vi "Main.vi"(11 "Module Admin":refnum<class "Delacor_lib_QMH_Module Admin.lvclass">) -> ()   [LabVIEW 2024, in "PLC.lvlib"]
doc: "This template is based off of the Queued Message Handler design pattern and the Queued Message Handler project template that ships with LabVIEW.\n\nThe main difference is that the queue is private to this module and communication between modules is performed via Broadcast and Request events.\n\nRequest events are wrapped in public API methods and are handled in the Event Handling Loop (EHL) of this VI. Any module can register for Broadcast events sent by this module. The EHL generates messages based on user interface actions.\n\nThe Message Handling Loop (MHL) processes messages generated by the EHL, or by other messages. The messages are string values, so new messages can be added easily to the Message Cases case structure in the MHL. Each message cluster can also provide an optional value for Message Data, which is a variant that can be converted to whatever message-specific data is required.\n_____\nBased on DQMH Dev Tools: Project Template 7.1.0.1503."
uses:
  PLC.lvlib
  <vilib>/Delacor/Delacor QMH/Libraries/Module Admin_class/Delacor_lib_QMH_Module Admin.lvclass
  Module Data--cluster.ctl
  <vilib>/Delacor/Delacor QMH/Libraries/Message Queue_class/Delacor_lib_QMH_Message Queue.lvclass/Delacor_lib_QMH_Message Queue.ctl
  Stop Argument--cluster.ctl
  <vilib>/Delacor/Delacor QMH/Libraries/Module Admin_class/Delacor_lib_QMH_Module Admin.lvclass/Delacor_lib_QMH_Module Admin.ctl
  set coil value Argument--cluster.ctl
  set register value Argument--cluster.ctl
  read coils Argument--cluster.ctl
  connect Argument--cluster.ctl
  <vilib>/Utility/miscctls.llb/LVPointTypeDef.ctl
  GUI/Controls/HW Modules.ctl
  <vilib>/Delacor/Delacor QMH/Libraries/Message Queue_class/Delacor_lib_QMH_Enqueue Message (Single).vi
  <vilib>/Delacor/Delacor QMH/Libraries/Module Admin_class/Delacor_lib_QMH_Get External Launch.vi
  <vilib>/NI/Modbus Library/API/Wrapper/Create TCP Master.vi
  <vilib>/Delacor/Delacor QMH/Libraries/Message Queue_class/Delacor_lib_QMH_Message Queue.lvclass
  <vilib>/NI/Modbus Library/API/Master/Modbus Master.lvclass
  <vilib>/NI/Modbus Library/API/Wrapper/API Main.lvlib
  GUI/GUI.lvlib
  Controller/Controller.lvlib
panel:
  out "coils":bool[](array[boolean])
  out "error out":errorcluster
  out "Status":string
  in  "Simulate MHL Error":bool
  in  "Simulate EHL Error":bool
  # "Other processes communicate with this Module via its Public API (wrappers for its Request Events).\n\nThis Module communicates with other processes via its Broadcast Events.\nAny process that wants to receive these messages can register for this module's Broadcast events."
  # "This template is for the DQMH framework. See the block diagram for more information on how to use this template."
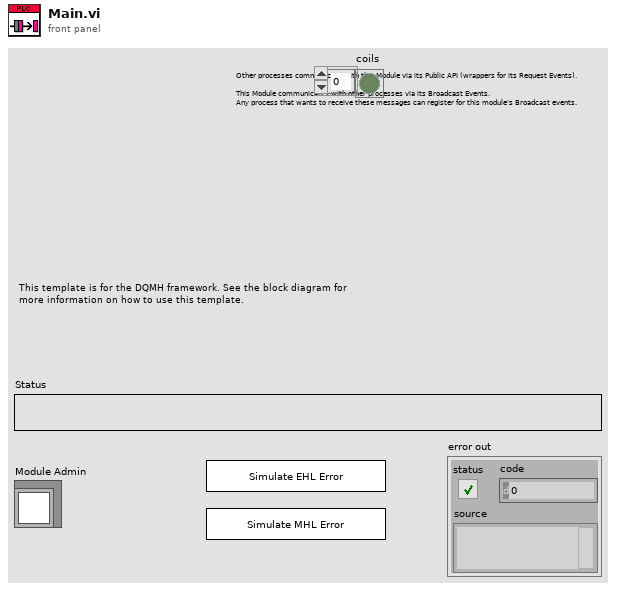
[diagram p1: front panel]
types:
  T1 = typedef "PLC.lvlib/Request Events--cluster.ctl" = cluster{"Stop Module":refnum<user-event>, "Show Panel":refnum<user-event>, "Hide Panel":refnum<user-event>, "Get Module Execution Status":refnum<user-event>, "Show Diagram":refnum<user-event>, "set coil value":refnum<user-event>, "set register value":refnum<user-event>, "Private.read coils":refnum<user-event>, "connect":refnum<user-event>}
  T2 = typedef "PLC.lvlib/Module Data--cluster.ctl" = cluster{"Status":string}
  T3 = enum32{"invalid lock state", "Not Locked", "Locked (No Password)", "Password-protected"}
  T4 = typedef "PLC.lvlib/Stop Argument--cluster.ctl" = cluster{"Origin":string, "Exit via Stop Module Req?":bool, "Wait for Module to stop?":bool}
  T5 = typedef "PLC.lvlib/set coil value Argument--cluster.ctl" = cluster{"ON/OFF":bool, "Ring":u16}
  T6 = typedef "PLC.lvlib/set register value Argument--cluster.ctl" = cluster{"Register number":u16, "value":dbl}
  T7 = typedef "PLC.lvlib/read coils Argument--cluster.ctl" = cluster{"number of coils to read":dbl}
  T8 = typedef "PLC.lvlib/connect Argument--cluster.ctl" = cluster{"IP address":string, "Port":dbl, "Flush events":bool}
  T9 = typedef "LVPointTypeDef.ctl" = cluster{"Horizontal":i16, "Vertical":i16}
  T10 = enum32{"Invalid", "Standard", "Closed", "Hidden", "Minimized", "Maximized"}
  T11 = typedef "HW Modules.ctl" = string
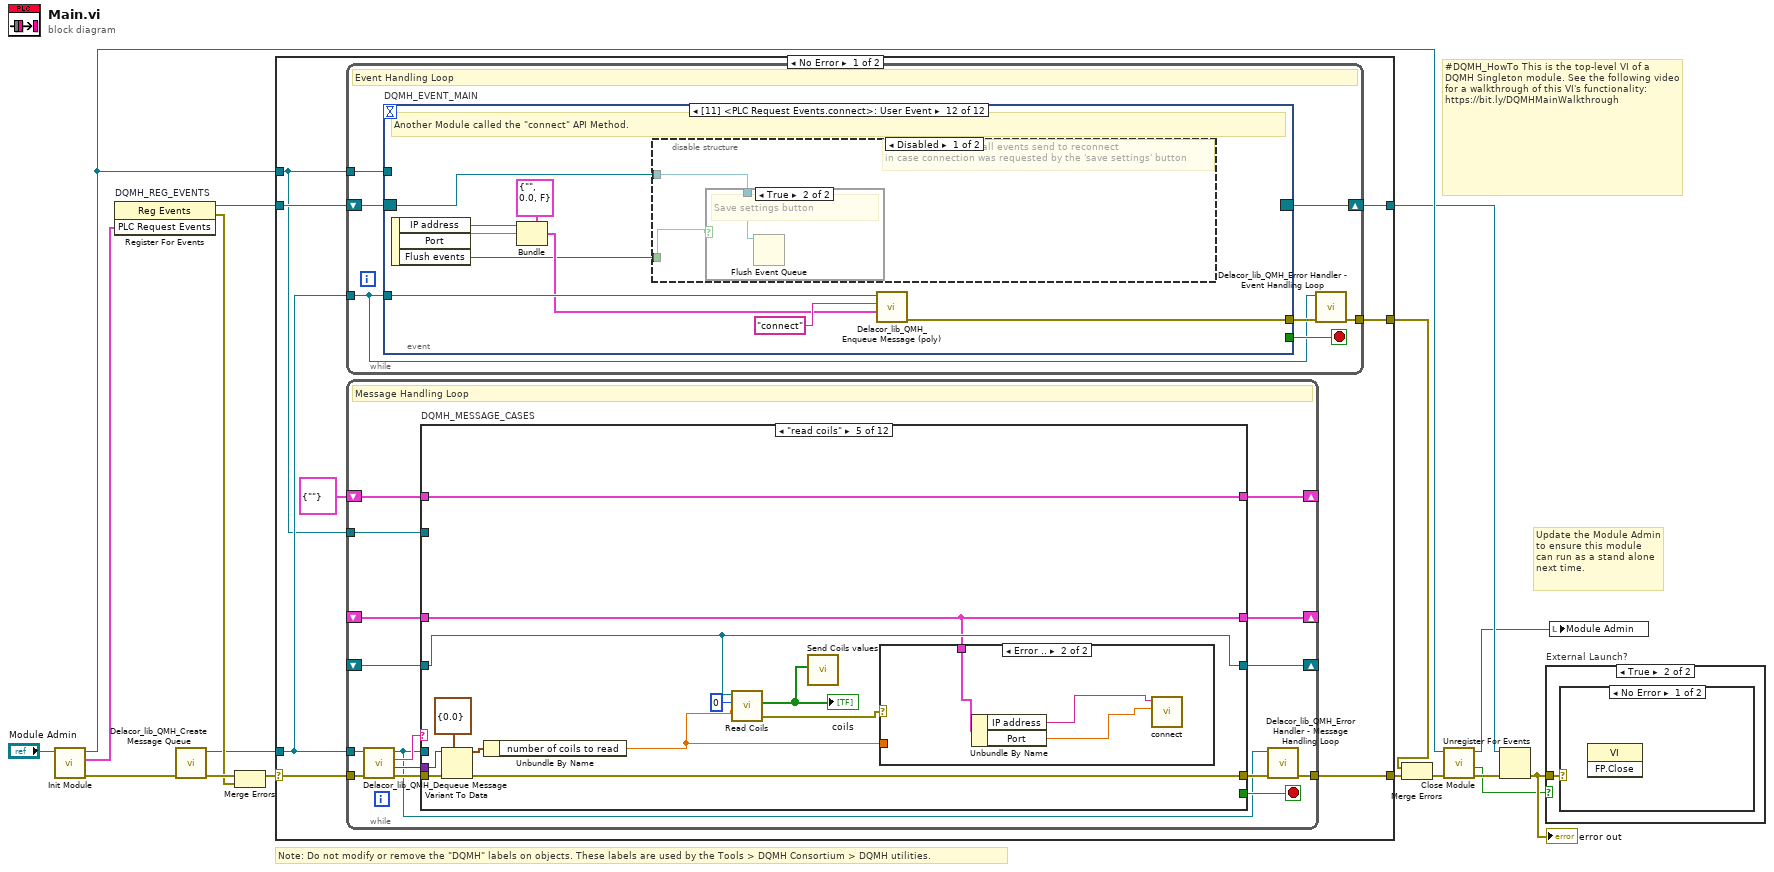
[diagram p0: block diagram]
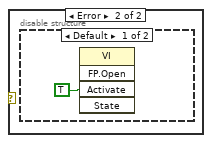
[diagram p3: hidden frame]
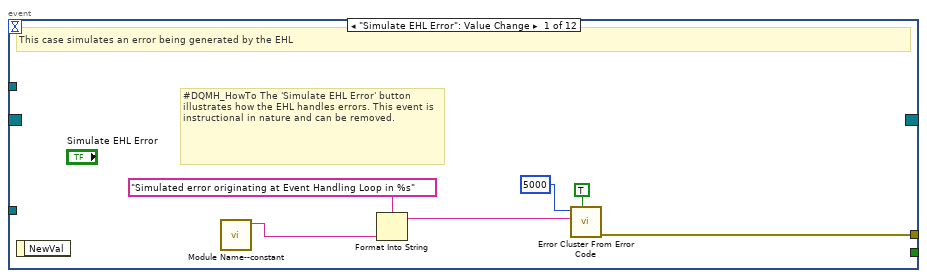
[diagram p5: hidden frame]
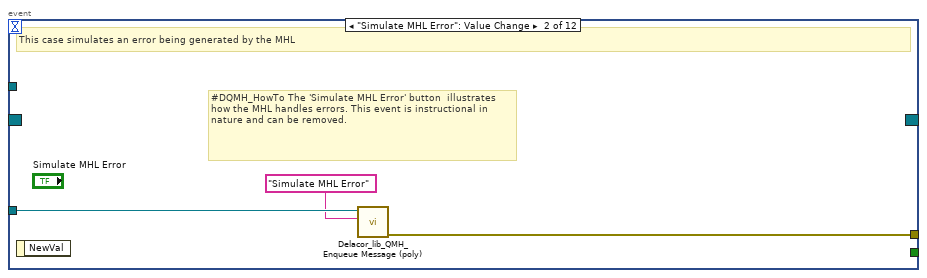
[diagram p6: hidden frame]
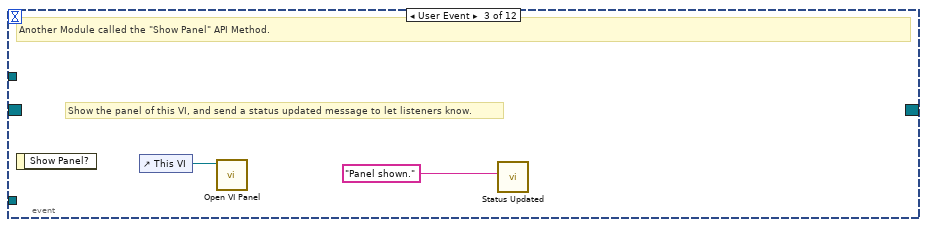
[diagram p7: hidden frame]
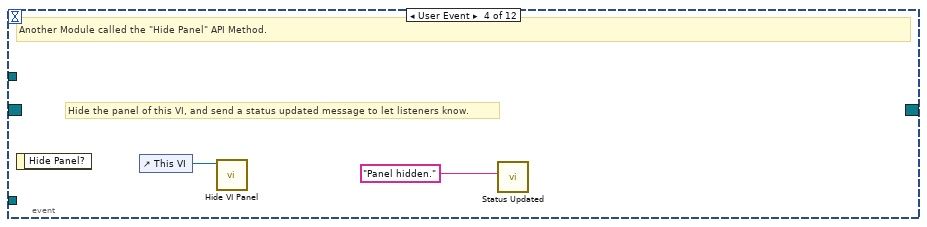
[diagram p8: hidden frame]
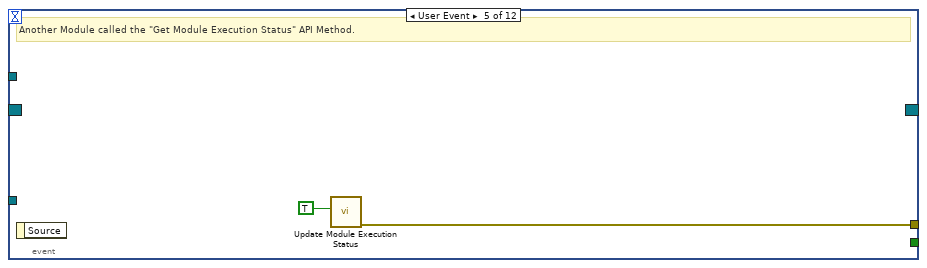
[diagram p9: hidden frame]
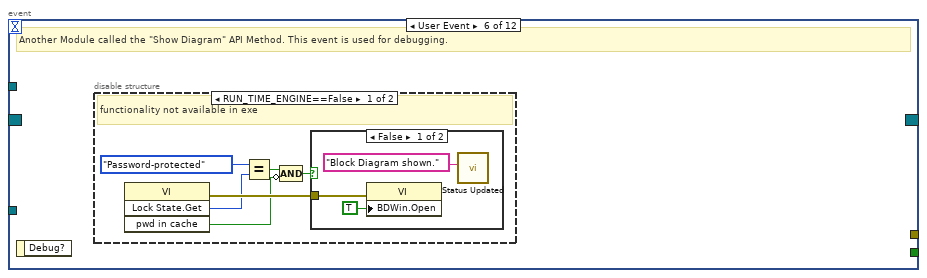
[diagram p10: hidden frame]
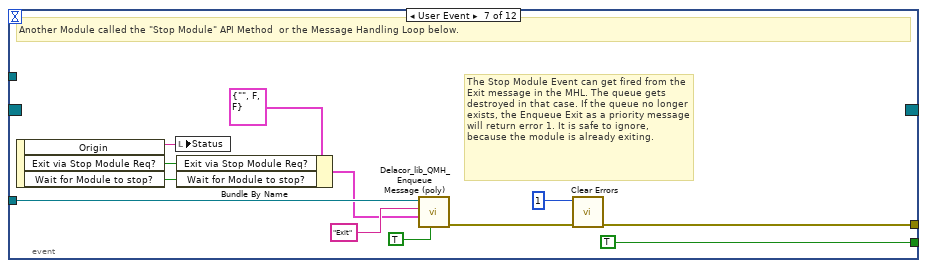
[diagram p13: hidden frame]
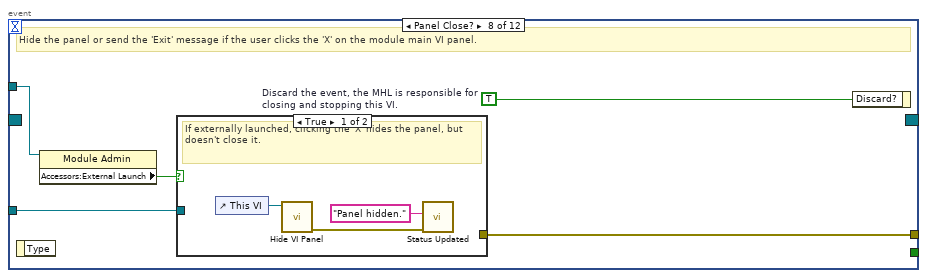
[diagram p14: hidden frame]
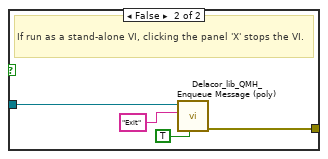
[diagram p15: hidden frame]
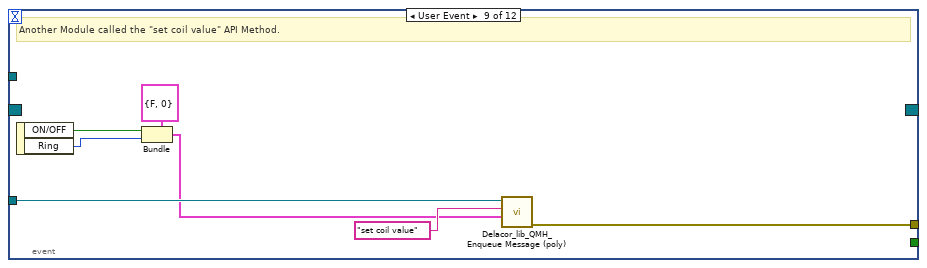
[diagram p16: hidden frame]
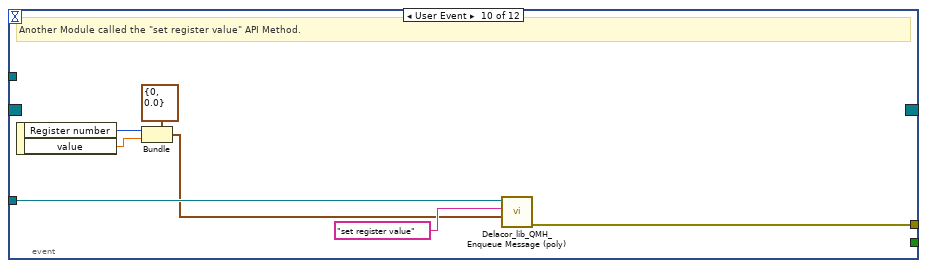
[diagram p17: hidden frame]
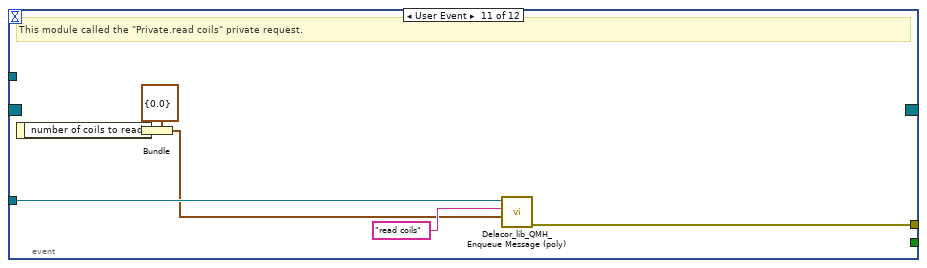
[diagram p18: hidden frame]
diagram:
  # "#DQMH_HowTo This is the top-level VI of a DQMH Singleton module. See the following video for a walkthrough of this VI's functionality: https://bit.ly/DQMHMainWalkthrough"
  # "Note: Do not modify or remove the \"DQMH\" labels on objects. These labels are used by the Tools > DQMH Consortium > DQMH utilities."
  # "Update the Module Admin to ensure this module can run as a stand alone next time."
  n1 = call "Init Module.vi"("Singleton Module Admin in"="Module Admin") -> ("error out"=w16:errorcluster, "PLC Request Events"=w5:T1, "Singleton Module Admin out"=w8:refnum<class "Delacor_lib_QMH_Module Admin.lvclass">)  [unwired: 8 in]
  n2 = register-events "DQMH_REG_EVENTS"(w5) -> (reference out=w6:refnum<event-registration>, error out=w9:errorcluster)  [unwired: 2 in]
  n3 = call <vilib>:"Delacor_lib_QMH_Create Message Queue.vi"("error in"=w16) -> ("error out"=w11:errorcluster, "Message Queue"=w4:refnum<class "Delacor_lib_QMH_Message Queue.lvclass">)  [unwired: 9 in]
  n4 = Merge Errors(w11, w9) -> (w10:errorcluster)
  n5 = case shown="No Error" w10 {
    selector: w10 -> [w23 w292]
    tunnel: [w25 w291] -> w17
    tunnel: [w22 w290] -> w7
    tunnel: w6 -> [w20 w290]
    tunnel: w4 -> [w19 w285]
    tunnel: [w24 _] -> w14
    tunnel: w8 -> [w18 w286]
    frame No Error {
      n6 = while {
        tunnel: w19 -> [w26]
        shift-right: [w29] -> w22
        shift-left: w20 -> [w30]
        tunnel: [w31] -> w24
        tunnel: w18 -> [w27]
        stop <- w28 stop-if-true
        # "Event Handling Loop"
        n7 = event "DQMH_EVENT_MAIN" shown="[11] <PLC Request Events.connect>: User Event" {
          selector: w30 -> [_ _ _ _ _ _ _ _ _ _ _ w102]
          dyn-events: [_ _ _ _ _ _ _ _ _ _ _ _] -> w29
          timeout: _ -> [_ _ _ _ _ _ _ _ _ _ _ _]
          tunnel: [_ _ _ _ _ _ TRUE ("Discard?") _ _ _ _ _] -> w28
          tunnel: w26 -> [_ w40 _ _ _ _ w64 w71 w87 w94 w100 w109]
          tunnel: [w38 w41 _ _ w47 _ w67 w73 w81 w88 w95 w103] -> w32
          tunnel: w27 -> [_ _ _ _ _ _ _ w70 _ _ _ _]
          event "Simulate EHL Error": Value Change {
            # "#DQMH_HowTo The 'Simulate EHL Error' button  illustrates how the EHL handles errors. This event is instructional in nature and can be removed."
            # "This case simulates an error being generated by the EHL"
            n8 = event-data() -> ()  [unwired: 1 in, 1 out]
            n9 = call "Module Name--constant.vi"() -> ("Module Name"=w35:string)  [unwired: 11 in]
            n10 = Format Into String(format string="Simulated error originating at Event Handling Loop in %s", w35) -> (resulting string=w36:string)  [unwired: 2 in, 1 out]
            n11 = call <vilib>:"Error Cluster From Error Code.vi"("show call chain? (False)"=TRUE, "error message (\"\")"=w36, "error code (0)"=5000) -> ("error out"=w38:errorcluster)  [unwired: 6 in]
          }
          event "Simulate MHL Error": Value Change {
            # "#DQMH_HowTo The 'Simulate MHL Error' button  illustrates how the MHL handles errors. This event is instructional in nature and can be removed."
            # "This case simulates an error being generated by the MHL"
            n12 = event-data() -> ()  [unwired: 1 in, 1 out]
            n13 = call-poly <vilib>:"Delacor_lib_QMH_Enqueue Message (poly).vi"("Message"="Simulate MHL Error", "Message Queue in"=w40) -> ("error out"=w41:errorcluster)  [unwired: 8 in, 1 out]
          }
          event User Event {
            # "Show the panel of this VI, and send a status updated message to let listeners know."
            # "Another Module called the \"Show Panel\" API Method."
            n14 = event-data() -> ()  [unwired: 1 in, 1 out]
            n15 = control-ref of="This VI"() -> (w43:refnum<vi>)
            n16 = call "Open VI Panel.vi"("VI"=w43) -> ()  [unwired: 10 in, 1 out]
            n17 = call "Status Updated.vi"("Status"="Panel shown." ("format string")) -> ()  [unwired: 10 in, 1 out]
          }
          event User Event {
            # "Hide the panel of this VI, and send a status updated message to let listeners know."
            # "Another Module called the \"Hide Panel\" API Method."
            n18 = event-data() -> ()  [unwired: 1 in, 1 out]
            n19 = control-ref of="This VI"() -> (w45:refnum<vi>)
            n20 = call "Hide VI Panel.vi"("VI"=w45) -> ()  [unwired: 10 in, 1 out]
            n21 = call "Status Updated.vi"("Status"="Panel hidden." ("format string")) -> ()  [unwired: 10 in, 1 out]
          }
          event User Event {
            # "Another Module called the \"Get Module Execution Status\" API Method."
            n22 = event-data() -> ()  [unwired: 1 in, 1 out]
            n23 = call "Update Module Execution Status.vi"("Running?"=TRUE) -> ("error out"=w47:errorcluster)  [unwired: 10 in]
          }
          event User Event {
            # "Another Module called the \"Show Diagram\" API Method. This event is used for debugging."
            n24 = event-data() -> ()  [unwired: 1 in, 1 out]
            n25 = disable-structure shown="RUN_TIME_ENGINE==False" {
              frame condition #0 (active) {
                # "functionality not available in exe"
                n26 = invoke on="Invoke Node" class="VI" method="Lock State.Get"() -> (error out=w53:errorcluster, "Get Lock State"=w52:T3, "pwd in cache"=w49:bool)  [unwired: 4 in, 1 out]
                n27 = Equal?(x=T3."Password-protected", y=w52) -> (x = y?=w50:bool)
                n28 = Compound Arithmetic op=AND(w50, invert w49) -> (w48:bool)
                n29 = case shown="False" w48 {
                  tunnel: w53 -> [w56 _]
                  frame False {
                    n30 = property on="Property Node" class="VI"(error in=w56, "BDWin.Open"=TRUE ("Block Diagram Window:Open")) -> ()  [unwired: 1 in, 2 out]
                    n31 = call "Status Updated.vi"("Status"="Block Diagram shown." ("format string")) -> ()  [unwired: 10 in, 1 out]
                  }
                  frame True {
                    # "Password-protected VI, and the password is not in the cache. Do not show the diagram."
                  }
                }
              }
              frame condition #1 {
              }
            }
          }
          event User Event {
            # "The Stop Module Event can get fired from the Exit message in the MHL. The queue gets destroyed in that case. If the queue no longer exists, the Enqueue Exit as a priority message will return error 1. It is safe to ignore, because the module is already exiting."
            # "Another Module called the \"Stop Module\" API Method  or the Message Handling Loop below."
            n32 = event-data() -> ("Origin"=w63:string, "Exit via Stop Module Req?"=w59:bool, "Wait for Module to stop?"=w58:bool)  [unwired: 1 in]
            n33 = local write "Status"(w63) -> ()
            n34 = Bundle By Name(cluster=T4 {"Origin"="", "Exit via Stop Module Req?"=FALSE, "Wait for Module to stop?"=FALSE} ("Stop Argument"), "Exit via Stop Module Req?"=w59, "Wait for Module to stop?"=w58) -> (w57:T4)
            n35 = call-poly <vilib>:"Delacor_lib_QMH_Enqueue Message (poly).vi"("Priority Message? (F)"=TRUE, "Message Data"=w57, "Message"="Exit", "Message Queue in"=w64) -> ("error out"=w68:errorcluster)  [unwired: 6 in, 1 out]
            n36 = call <vilib>:"Clear Errors.vi"("error in (no error)"=w68, "specific error code to clear (0: all)"=1) -> ("error out"=w67:errorcluster)  [unwired: 4 in, 1 out]
          }
          event Panel Close? {
            w72 = TRUE  # Discard the event, the MHL is responsible for closing and stopping this VI.
            # "Hide the panel or send the 'Exit' message if the user clicks the 'X' on the module main VI panel."
            n37 = event-data() -> ()  [unwired: 1 in, 1 out]
            n38 = property on="Property Node" class="Module Admin"(reference=w70) -> ("Accessors:External Launch"=w69:bool)  [unwired: 1 in, 2 out]
            n39 = case shown="True" w69 {
              tunnel: w71 -> [_ w79]
              tunnel: [_ w80] -> w73
              frame True {
                # "If externally launched, clicking the 'X' hides the panel, but doesn't close it."
                n40 = control-ref of="This VI"() -> (w76:refnum<vi>)
                n41 = call "Hide VI Panel.vi"("VI"=w76) -> ("error out"=w74:errorcluster)  [unwired: 10 in]
                n42 = call "Status Updated.vi"("error in"=w74, "Status"="Panel hidden." ("format string")) -> ()  [unwired: 9 in, 1 out]
              }
              frame False {
                # "If run as a stand-alone VI, clicking the panel 'X' stops the VI."
                n43 = call-poly <vilib>:"Delacor_lib_QMH_Enqueue Message (poly).vi"("Priority Message? (F)"=TRUE, "Message"="Exit", "Message Queue in"=w79) -> ("error out"=w80:errorcluster)  [unwired: 7 in, 1 out]
              }
            }
            n44 = event-data ("Event Filter Node")("Discard?"=w72) -> ()  [unwired: 1 in, 1 out]
          }
          event User Event {
            # "Another Module called the \"set coil value\" API Method."
            n45 = event-data() -> ("ON/OFF"=w83:bool, "Ring"=w82:u16)  [unwired: 1 in]
            n46 = Bundle(cluster=T5 {"ON/OFF"=FALSE, "Ring"=0} ("set coil value Argument"), "ON/OFF"=w83, "Ring"=w82) -> (w84:T5)
            n47 = call-poly <vilib>:"Delacor_lib_QMH_Enqueue Message (poly).vi"("Message Data"=w84, "Message"="set coil value", "Message Queue in"=w87) -> ("error out"=w81:errorcluster)  [unwired: 7 in, 1 out]
          }
          event User Event {
            # "Another Module called the \"set register value\" API Method."
            n48 = event-data() -> ("Register number"=w90:u16, "value"=w89:dbl)  [unwired: 1 in]
            n49 = Bundle(cluster=T6 {"Register number"=0, "value"=0.0} ("set register value Argument"), "Register number"=w90, "value"=w89) -> (w91:T6)
            n50 = call-poly <vilib>:"Delacor_lib_QMH_Enqueue Message (poly).vi"("Message Data"=w91, "Message"="set register value", "Message Queue in"=w94) -> ("error out"=w88:errorcluster)  [unwired: 7 in, 1 out]
          }
          event User Event {
            # "This module called the \"Private.read coils\" private request."
            n51 = event-data() -> ("number of coils to read"=w96:dbl)  [unwired: 1 in]
            n52 = Bundle(cluster=T7 {"number of coils to read"=0.0} ("read coils Argument"), "number of coils to read"=w96) -> (w97:T7)
            n53 = call-poly <vilib>:"Delacor_lib_QMH_Enqueue Message (poly).vi"("Message Data"=w97, "Message"="read coils", "Message Queue in"=w100) -> ("error out"=w95:errorcluster)  [unwired: 7 in, 1 out]
          }
          event User Event {
            # "Another Module called the \"connect\" API Method."
            n54 = event-data() -> ("IP address"=w105:string, "Port"=w104:dbl, "Flush events"=w101:bool)  [unwired: 1 in]
            n55 = Bundle(cluster=T8 {"IP address"="", "Port"=0.0, "Flush events"=FALSE} ("connect Argument"), "IP address"=w105, "Port"=w104) -> (w106:T8)  [unwired: 1 in]
            n56 = disable-structure shown="Disabled" {
              disable-tunnel: w102 -> [w111 _]
              disable-tunnel: w101 -> [w110 _]
              frame Disabled {
                # "this is used to flush all events send to reconnect\nin case connection was requested by the 'save settings' button"
                n57 = case shown="True" w110 {
                  tunnel: w111 -> [_ w112]
                  frame False {
                    # "reconnect by the same module"
                  }
                  frame True {
                    # "Save settings button"
                    n58 = Flush Event Queue(0:w112) -> ()  [unwired: 5 in, 3 out]
                  }
                }
              }
              frame Enabled {
              }
            }
            n59 = call-poly <vilib>:"Delacor_lib_QMH_Enqueue Message (poly).vi"("Message Data"=w106, "Message"="connect", "Message Queue in"=w109) -> ("error out"=w103:errorcluster)  [unwired: 7 in, 1 out]
          }
        }
        n60 = call-dynamic "Delacor_lib_QMH_Error Handler - Event Handling Loop.vi"("error in"=w32, "Message Queue in"=w26) -> ("dup error in"=w31:errorcluster)  [unwired: 8 in, 1 out]
      }
      n61 = while {
        tunnel: w19 -> [w117]
        shift-right: [w125] -> _
        shift-left: T2 {"Status"=""} ("Data Cluster") -> [w126]
        tunnel: w23 -> [w128]
        tunnel: [w120] -> w25
        tunnel: w18 -> [w121]
        shift-right: [w116] -> _
        shift-left: _ -> [w115]
        shift-right: [w114] -> _
        shift-left: _ -> [w113]
        stop <- w124 stop-if-true
        # "Message Handling Loop"
        n62 = call-dynamic "Delacor_lib_QMH_Dequeue Message.vi"("error in"=w128, "Message Queue in"=w117) -> ("error out"=w127:errorcluster, "Message Data"=w122:variant, "Message"=w123:string, "Message Queue out"=w118:refnum<class "Delacor_lib_QMH_Message Queue.lvclass">)  [unwired: 6 in]
        n63 = case "DQMH_MESSAGE_CASES" shown="\"read coils\"" w123 {
          selector: w123 -> [_ _ _ _ _ _ _ _ _ _ _ w280]
          tunnel: w118 -> [_ _ _ _ _ w189 _ _ _ w242 w266 _]
          tunnel: w127 -> [w148 w154 w162 w170 w182 w205 w221 w225 w236 w249 w272 w283]
          tunnel: [w146 w154 w160 w168 w180 w203 w220 w225 w235 w245 w267 w284] -> w119
          tunnel: w126 -> [w137 w153 w161 w169 w181 w204 w219 w224 w233 w244 w265 w281]
          tunnel: [w136 w153 w161 w169 w181 w204 w219 w224 w233 w244 w265 w281] -> w125
          tunnel: [_ _ _ _ _ _ _ _ _ _ w264 _] -> w124
          tunnel: w122 -> [_ _ w159 w167 w179 w202 _ _ _ w243 w263 _]
          tunnel: w121 -> [w138 _ _ _ _ _ _ _ _ w241 w258 _]
          tunnel: [w130 w152 w156 w164 w176 w199 w218 w223 w227 w238 w257 w274] -> w116
          tunnel: w115 -> [w130 w152 w156 w164 w176 w192 w218 w223 w227 w238 w257 w274]
          tunnel: [w129 w151 w155 w163 w173 w195 w217 w222 w226 w237 w256 w273] -> w114
          tunnel: w113 -> [w129 w151 w155 w163 w173 _ w217 w222 w226 w237 w256 w273]
          frame "Initialize" {
            w132 = "Initial Message" ("Initial Message")
            # "#DQMH_CodeNeeded - Initialize the appearance of the front panel."
            # "#DQMH_CodeNeeded - Initialize your state data here."
            # "Initialize - Any operation that needs to be done before the module can receive messages. Synchronize Caller Events.vi will inform Start Module.vi that the module has launched and is ready to receive messages. Module Did Init.vi will broadcast that the module initialized."
            n64 = call "Synchronize Caller Events.vi"("error in"=w148, "Singleton Module Admin in"=w138) -> ("error out"=w147:errorcluster, "Singleton Module Admin out"=w133:refnum<class "Delacor_lib_QMH_Module Admin.lvclass">)  [unwired: 8 in]
            n65 = property on="Property Node" class="Module Admin"(reference=w133) -> ("Accessors:External Launch"=w142:bool)  [unwired: 1 in, 2 out]
            n66 = Select(t=T10."Hidden" ("State"), s=w142, f=T10."Standard" ("State")) -> (s? t:f=w139:T10)
            n67 = call "Module Name--constant.vi"() -> ("Module Name"=w145:string)  [unwired: 11 in]
            n68 = property on="Property Node" class="VI"("Front Panel.Title"=w145) -> (reference out=w144:refnum<vi>, error out=w150:errorcluster)  [unwired: 2 in]
            n69 = invoke on="Invoke Node" class="VI" method="FP.Open"(reference=w144, error in=w150, "State"=w139) -> (reference out=w143:refnum<vi>, error out=w149:errorcluster)  [unwired: 2 in, 3 out]
            n70 = Bundle By Name(cluster=w137, "Status"=w132) -> (w136:T2)
            n71 = invoke on="Invoke Node" class="VI" method="FP.Center"(reference=w143, error in=w149) -> ()  [unwired: 1 in, 3 out]
            n72 = property on="Pane" class="Pane"("Origin"=T9 {"Horizontal"=0, "Vertical"=0}) -> ()  [unwired: 2 in, 2 out]
            n73 = call "Module Name--constant.vi"() -> ("Module Name"=w134:string)  [unwired: 11 in]
            n74 = call "Module Did Init.vi"("error in"=w147, "Initialized?"=TRUE, "Origin"=w134) -> ("error out"=w146:errorcluster)  [unwired: 8 in]
            "Status" <- w132
          }
          frame "---Module Specific---" {
            # "Separator -- The following cases handle messages specific to this Module."
          }
          frame "set coil value" {
            # "#DQMH_CodeNeeded\n1. Configure this Message Case for handling the \"set coil value\" message.\n2. Delete or edit this label when done."
            n75 = Variant To Data(error in=w162, type=T5 {"ON/OFF"=FALSE, "Ring"=0} ("set coil value Argument"), Variant=w159) -> (data=w157:T5, error out=w160:errorcluster)
            n76 = Unbundle By Name(w157) -> ()  [unwired: 2 out]
          }
          frame "set register value" {
            # "#DQMH_CodeNeeded\n1. Configure this Message Case for handling the \"set register value\" message.\n2. Delete or edit this label when done."
            n77 = Variant To Data(error in=w170, type=T6 {"Register number"=0, "value"=0.0} ("set register value Argument"), Variant=w167) -> (data=w165:T6, error out=w168:errorcluster)
            n78 = Unbundle By Name(w165) -> ()  [unwired: 2 out]
          }
          frame "read coils" {
            n79 = Variant To Data(error in=w182, type=T7 {"number of coils to read"=0.0} ("read coils Argument"), Variant=w179) -> (data=w177:T7, error out=w180:errorcluster)
            n80 = Unbundle By Name(w177) -> ("number of coils to read"=w172:dbl)
            n81 = call-dynamic "Read Coils.vi"("number of inputs"=w172, "starting address"=u16 0, "Modbus master in"=w176) -> ("error out"=w174:errorcluster, "coils"=w171:bool[])  [unwired: 6 in, 1 out]
            "coils" <- w171
            n82 = call "Send Coils values.vi"("Coils"=w171) -> ()  [unwired: 10 in, 1 out]
            n83 = case shown="Error .." w174 {
              tunnel: w173 -> [_ w187]
              tunnel: w172 -> [w183 _]
              frame No Error {
                n84 = Wait (ms)(milliseconds to wait=u32 20) -> ()  [unwired: 1 out]
                n85 = call "read coils.vi"("number of coils to read"=w183) -> ()  [unwired: 10 in, 1 out]
              }
              frame Error {
                n86 = Unbundle By Name(w187) -> ("IP address"=w186:string, "Port"=w185:dbl)
                n87 = call "connect.vi"("Port"=w185, "IP address"=w186) -> ()  [unwired: 9 in, 1 out]
              }
            }
          }
          frame "connect" {
            n88 = Variant To Data(error in=w205, type=T8 {"IP address"="", "Port"=0.0, "Flush events"=FALSE} ("connect Argument"), Variant=w202) -> (data=w195:T8, error out=w203:errorcluster)
            n89 = Unbundle By Name(w195) -> ("IP address"=w197:string, "Port"=w196:dbl)
            n90 = call-dynamic "Delacor_lib_QMH_Flush Messages.vi"("Message Queue in"=w189) -> ("error out"=w188:errorcluster)  [unwired: 7 in, 3 out]
            n91 = call-dynamic "Shutdown.vi"("error in"=w188, "Modbus master in"=w192) -> ("error out"=w191:errorcluster)  [unwired: 9 in]
            n92 = call <vilib>:"Clear Errors.vi"("error in (no error)"=w191) -> ("error out"=w190:errorcluster)  [unwired: 5 in, 1 out]
            n93 = call-poly <vilib>:"Create Modbus Instance.vi"("error in"=w190, "connect timeout ms"=2000, "port (502)"=w196, "address"=w197) -> ("error out"=w198:errorcluster, "TCP master instance"=w199:refnum<class "Modbus Master.lvclass">)  [unwired: 6 in]
            n94 = case shown="No Error" w198 {
              tunnel: w197 -> [_ w214]
              tunnel: w196 -> [_ w213]
              tunnel: [TRUE FALSE] -> w194
              frame No Error {
                # "number of coils to\nread"
                n95 = call "read coils.vi"("number of coils to read"=2.0) -> ()  [unwired: 10 in, 1 out]
              }
              frame Error {
                n96 = Wait (ms)(milliseconds to wait=u32 10) -> ()  [unwired: 1 out]
                n97 = call "connect.vi"("Flush events"=FALSE, "Port"=w213, "IP address"=w214) -> ()  [unwired: 8 in, 1 out]
              }
            }
            n98 = disable-structure shown="Enabled" {
              disable-tunnel: w194 -> [w207 w208 _]
              disable-tunnel: T11 "PLC" ("HW Module") -> [w206 w209 _]
              frame Disabled {
                n99 = call "update HW status indicator.vi"("Status"=w207, "HW Module"=w206) -> ()  [unwired: 9 in, 1 out]
              }
              frame Enabled {
                n100 = call "HW Starus.vi"("Status"=w208, "HW Module"=w209) -> ()  [unwired: 9 in, 1 out]
              }
              frame Disabled {
              }
            }
          }
          frame "---Copy This Frame---" {
            # "Duplicate this frame when creating new messages.  Change this comment in the duplicated frame to describe this message."
            n101 = Merge Errors(w221) -> (w220:errorcluster)
          }
          frame "---Exit and Error Handling---" {
            # "Separator - The following cases handle errors and exit messages."
          }
          frame "Simulate MHL Error" {
            # "#DQMH_HowTo The 'Simulate MHL Error' button  illustrates how the MHL handles errors. This event is instructional in nature and can be removed."
            # "Simulate an error occurring at the MHL"
            n102 = call "Module Name--constant.vi"() -> ("Module Name"=w229:string)  [unwired: 11 in]
            n103 = Format Into String(format string="Simulated error originating at Message Handling Loop in %s", w229) -> (resulting string=w230:string)  [unwired: 2 in, 1 out]
            n104 = call <vilib>:"Error Cluster From Error Code.vi"("show call chain? (False)"=TRUE, "error message (\"\")"=w230, "error code (0)"=5001) -> ("error out"=w234:errorcluster)  [unwired: 6 in]
            n105 = Merge Errors(w236, w234) -> (w235:errorcluster)
          }
          frame "Error" {
            # "#DQMH_CodeRecommended - If the module is running in standalone mode (External Launch = FALSE), this code will pop up an error dialog and call the 'Exit' message if an error occurs. Add more fine-grained error management here."
            # "Error - Check the error message data and respond accordingly. This message is sent by the \"Error Handler\" VIs at the end of each loop in this application."
            n106 = property on="Property Node" class="Module Admin"(reference=w241) -> ("Accessors:External Launch"=w240:bool)  [unwired: 1 in, 2 out]
            n107 = Variant To Data(error in=w249, type=errorcluster {"status"=FALSE, "code"=0, "source"=""} ("error constant"), Variant=w243) -> (data=w239:errorcluster, error out=w247:errorcluster)
            n108 = local write "error out"(w239) -> ()
            n109 = call "Error Reported.vi"("Error"=w239) -> ()  [unwired: 10 in, 1 out]
            n110 = case shown="False" w240 {
              tunnel: [w254 _] -> w246
              tunnel: w242 -> [w252 _]
              tunnel: w239 -> [w253 _]
              frame False {
                n111 = disable-structure shown="Default" {
                  disable-tunnel: w253 -> [w255 _]
                  frame condition #0 (active) {
                    # "If the module is running standalone, then pop up an error dialog and call the \"Exit\" message."
                    n112 = call <vilib>:"Simple Error Handler.vi"("error in (no error)"=w255) -> ()  [unwired: 4 in, 5 out]
                  }
                  frame condition #1 {
                    # "To prevent the Simple Error Handler VI from being loaded (e.g. when deploying to a Real-Time target), add the Conditional Disable Symbol \"DQMH_Disable_SEH\" to your project and set it to TRUE."
                  }
                }
                n113 = call-poly <vilib>:"Delacor_lib_QMH_Enqueue Message (poly).vi"("Priority Message? (F)"=TRUE, "Message"="Exit", "Message Queue in"=w252) -> ("error out"=w254:errorcluster)  [unwired: 7 in, 1 out]
              }
              frame True {
                # "If the module was launched externally, calling the Error Reported broadcast VI is the only action performed by the \"Error\" message. The module's caller can then process the error appropriately."
              }
            }
            n114 = Merge Errors(w247, w246) -> (w245:errorcluster)
          }
          frame "Exit" {
            w262 = 91  # 91: not all Exit messages will have an argument
            w264 = TRUE  # Stop the VI
            # "Release the message queue reference"
            # "#DQMH_CodeNeeded - Add any required cleanup code here."
            # "Exit - Exit the application."
            n115 = Variant To Data(error in=w272, type=T4 {"Origin"="", "Exit via Stop Module Req?"=FALSE, "Wait for Module to stop?"=FALSE} ("Stop Argument"), Variant=w263) -> (data=w260:T4, error out=w269:errorcluster)
            n116 = call <vilib>:"Clear Errors.vi"("error in (no error)"=w269, "specific error code to clear (0: all)"=w262) -> ("error out"=w271:errorcluster)  [unwired: 4 in, 1 out]
            n117 = control-ref of="This VI"() -> (w259:refnum<vi>)
            n118 = call-dynamic "Delacor_lib_QMH_Release Message Queue.vi"("error in"=w271, "Message Queue"=w266) -> ("error out"=w270:errorcluster)  [unwired: 9 in]
            n119 = call "Handle Exit.vi"("Stop Argument"=w260, "Admin in"=w258, "VI reference"=w259) -> ("error out"=w268:errorcluster)  [unwired: 7 in, 1 out]
            n120 = Merge Errors(w270, w268) -> (w267:errorcluster)
            n121 = call "Error Reported.vi"("Error"=w267) -> ()  [unwired: 10 in, 1 out]
          }
          frame Default {
            # "'Default' case only runs if there is a message that isn't defined in any of the other cases.  Output a programming error."
            n122 = call "Module Name--constant.vi"() -> ("Module Name"=w279:string)  [unwired: 11 in]
            n123 = Format Into String(format string="The invalid message string \"%s\" was received in the Message Handling Loop for module \"%s\".", w280, w279) -> (resulting string=w275:string)  [unwired: 2 in, 1 out]
            n124 = call <vilib>:"Error Cluster From Error Code.vi"("show call chain? (False)"=TRUE, "error message (\"\")"=w275, "error code (0)"=1) -> ("error out"=w282:errorcluster)  [unwired: 6 in]
            n125 = Merge Errors(w283, w282) -> (w284:errorcluster)
          }
        }
        n126 = call-dynamic "Delacor_lib_QMH_Error Handler - Message Handling Loop.vi"("error in"=w119, "Message Queue in"=w118) -> ("dup error in"=w120:errorcluster)  [unwired: 8 in, 1 out]
      }
    }
    frame Error {
      # "Synchronize Caller Events.vi will inform Start Module.vi that the module has launched and will let the code calling Start Module.vi register for broadcasts and would permit the caller receive the broadcast that an error occurred at launch time."
      n127 = call-dynamic "Delacor_lib_QMH_Release Message Queue.vi"("error in"=w292, "Message Queue"=w285) -> ("error out"=w291:errorcluster)  [unwired: 9 in]
      n128 = call "Synchronize Caller Events.vi"("Singleton Module Admin in"=w286) -> ("error out"=w293:errorcluster)  [unwired: 9 in, 1 out]
      n129 = call "Module Name--constant.vi"() -> ("Module Name"=w289:string)  [unwired: 11 in]
      n130 = Format Into String(format string="An error occurred during initialization. %s is no longer running.", w289) -> (resulting string=w287:string)  [unwired: 2 in, 1 out]
      n131 = Merge Errors(w291, w293) -> (w294:errorcluster)
      n132 = call "Error Reported.vi"("Additional Information"=w287, "Error"=w294) -> ()  [unwired: 9 in, 1 out]
    }
  }
  n133 = Merge Errors(w14, w17) -> (w13:errorcluster)
  n134 = call "Close Module.vi"("error in"=w13, "Module Admin in"=w8) -> ("error out"=w15:errorcluster, "External Launch"=w1:bool, "Module Admin out"=w2:refnum<class "Delacor_lib_QMH_Module Admin.lvclass">)  [unwired: 7 in]
  n135 = Unregister For Events(event registration refnum=w7, error in=w15) -> (error out=w12:errorcluster)
  "error out" <- w12
  n136 = case "External Launch?" shown="True" w1 {
    tunnel: w12 -> [_ w295]
    frame False {
    }
    frame True {
      n137 = case shown="No Error" w295 {
        frame No Error {
          n138 = invoke on="Invoke Node" class="VI" method="FP.Close"() -> ()  [unwired: 3 in, 3 out]
        }
        frame Error {
          n139 = disable-structure shown="Default" {
            frame condition #0 (active) {
              n140 = invoke class="VI" method="FP.Open"("Activate"=TRUE ("Activate?")) -> ()  [unwired: 4 in, 5 out]
            }
            frame condition #1 {
              # "Don't show panel on error if running inside a built EXE."
            }
          }
        }
      }
    }
  }
  n141 = local write "Module Admin"(w2) -> ()
